vi "Construct Scanner.vi"(11 "Scanner Enum In":T1) -> (0 "error out":errorcluster, 3 "Scanner out":refnum<class "Scanner.lvclass">)   [LabVIEW 2017, in "Scan Driver.lvclass"]
uses:
  Scan Driver.lvclass
  Scanner List.ctl
  Scanners/Scanner/Scanner.lvclass
  Scanners/Dummy Scan/Dummy Scan.lvclass
  C:/LabVIEW-programs/Scanners/Scanner/Scanner.lvclass
  Scanners/Magnetic Field Lakeshore Continuous/Magnetic Field Lakeshore Continuous.lvclass
  Scanners/Magnetic Field Oxford Continuous/Magnetic Field Oxford Continuous.lvclass
  Instruments/Analog Output/Analog Output.lvclass
  Instruments/Function Generator/Function Generator.lvclass
  Instruments/Lakeshore Gaussmeter/Lakeshore Gaussmeter.lvclass
  Instruments/Oxford Magnet/Power Supply/Power Supply.lvclass
  Instruments/Magna-Power Power Supply/Magna Power.lvclass
  Instruments/Microwave/Microwave.lvclass
  Instruments/Pulse Gen/Pulse Generator.lvclass
  Instruments/Translation Stages/Translation Stages.lvclass
  Instruments/Spectrometer/Spectrometer Triax 550.lvclass
  Instruments/Spectrometer ActiveX/Spectrometer ActiveX.lvclass
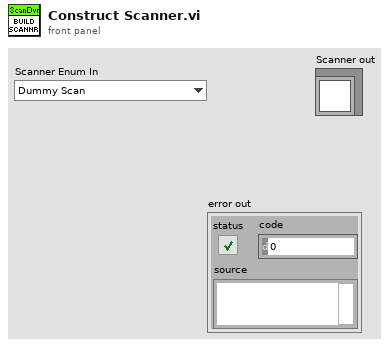
[diagram p1: front panel]
types:
  T1 = typedef "Scan Driver.lvclass/Scanner List.ctl" = enum16{"Dummy Scan", "Analog Output Scan", "Function Gen Scan", "Magnetic Field Lakeshore", "Magnetic Field Lakeshore Continuous", "Magnetic Field Oxford", "Magnetic Field Oxford Continuous", "Magna Current Scan", "Magna Voltage Scan", "Microwave Freq Scan", "Pulse Gen Scan", "Pulse Gen Basic Scan", "Translation Stage Dual", "Translation Stage Coarse", "Translation Stage Fine", "Wavelength", "Wavelength Digikröm", "Wavelength ActiveX", "None"}
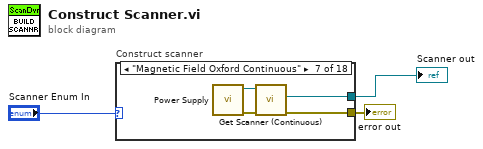
[diagram p0: block diagram]
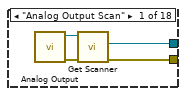
[diagram p2: hidden frame]
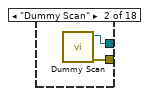
[diagram p3: hidden frame]
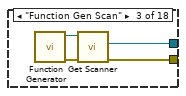
[diagram p4: hidden frame]
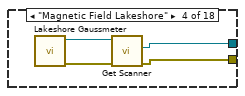
[diagram p5: hidden frame]
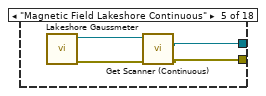
[diagram p6: hidden frame]
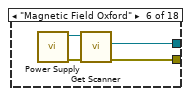
[diagram p7: hidden frame]
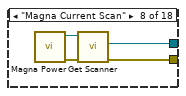
[diagram p8: hidden frame]
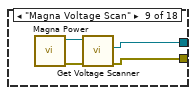
[diagram p9: hidden frame]
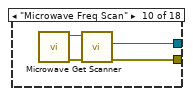
[diagram p10: hidden frame]
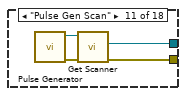
[diagram p11: hidden frame]
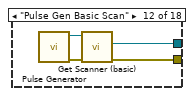
[diagram p12: hidden frame]
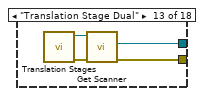
[diagram p13: hidden frame]
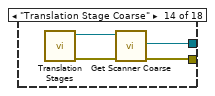
[diagram p14: hidden frame]
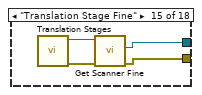
[diagram p15: hidden frame]
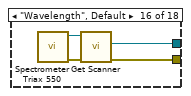
[diagram p16: hidden frame]
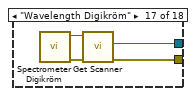
[diagram p17: hidden frame]
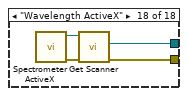
[diagram p18: hidden frame]
diagram:
  n1 = case "Construct scanner" shown="\"Magnetic Field Oxford Continuous\"" "Scanner Enum In" {
    tunnel: [w4 w9 w12 w14 w20 w24 w28 w31 w35 w40 w44 w47 w52 w54 w59 w64 w68 w70] -> w2
    tunnel: [w5 w8 w10 w15 w18 w22 w26 w30 w34 w38 w42 w46 w50 w55 w58 w63 w66 w71] -> w3
    frame "Analog Output Scan" {
      n2 = call "Analog Output.vi"() -> ("error out"=w6:errorcluster, "Analog Output out"=w7:refnum<class "Analog Output.lvclass">)  [unwired: 10 in]
      n3 = call-dynamic "Get Scanner.vi"("error in (no error)"=w6, "Analog Output in"=w7) -> ("error out"=w5:errorcluster, "Default Scanner out"=w4:refnum<class "Scanner.lvclass">)  [unwired: 8 in]
    }
    frame "Dummy Scan" {
      n4 = call "Dummy Scan.vi"() -> ("error out"=w8:errorcluster, "Dummy Scan out"=w9:refnum<class "Dummy Scan.lvclass">)  [unwired: 10 in]
    }
    frame "Function Gen Scan" {
      n5 = call "Function Generator.vi"() -> ("error out"=w11:errorcluster, "Function Generator out"=w13:refnum<class "Function Generator.lvclass">)  [unwired: 1 in, 9 out]
      n6 = call-dynamic "Get Scanner.vi"("error in (no error)"=w11, "Function Generator in"=w13) -> ("error out"=w10:errorcluster, "Default Scanner out"=w12:refnum<class "Scanner.lvclass">)  [unwired: 8 out]
    }
    frame "Magnetic Field Lakeshore" {
      n7 = call "Lakeshore Gaussmeter.vi"() -> ("error out"=w16:errorcluster, "Lakeshore Gaussmeter out"=w17:refnum<class "Lakeshore Gaussmeter.lvclass">)  [unwired: 10 in]
      n8 = call-dynamic "Get Scanner.vi"("error in (no error)"=w16, "Lakeshore Gaussmeter in"=w17) -> ("error out"=w15:errorcluster, "Default Scanner out"=w14:refnum<class "Scanner.lvclass">)  [unwired: 8 in]
    }
    frame "Magnetic Field Lakeshore Continuous" {
      n9 = call "Lakeshore Gaussmeter.vi"() -> ("error out"=w19:errorcluster, "Lakeshore Gaussmeter out"=w21:refnum<class "Lakeshore Gaussmeter.lvclass">)  [unwired: 10 in]
      n10 = call-dynamic "Get Scanner (Continuous).vi"("error in (no error)"=w19, "Lakeshore Gaussmeter in"=w21) -> ("error out"=w18:errorcluster, "Magnetic Field Lakeshore Continuous.lvclass out"=w20:refnum<class "Magnetic Field Lakeshore Continuous.lvclass">)  [unwired: 8 in]
    }
    frame "Magnetic Field Oxford" {
      n11 = call "Power Supply.vi"() -> ("error out"=w23:errorcluster, "Power Supply out"=w25:refnum<class "Power Supply.lvclass">)  [unwired: 10 in]
      n12 = call-dynamic "Get Scanner.vi"("error in (no error)"=w23, "Power Supply in"=w25) -> ("error out"=w22:errorcluster, "Default Scanner out"=w24:refnum<class "Scanner.lvclass">)  [unwired: 8 out]
    }
    frame "Magnetic Field Oxford Continuous" {
      n13 = call "Power Supply.vi"() -> ("error out"=w27:errorcluster, "Power Supply out"=w29:refnum<class "Power Supply.lvclass">)  [unwired: 10 in]
      n14 = call "Get Scanner (Continuous).vi"("error in (no error)"=w27, "Power Supply in"=w29) -> ("error out"=w26:errorcluster, "Continuous Scanner out"=w28:refnum<class "Magnetic Field Oxford Continuous.lvclass">)  [unwired: 8 in]
    }
    frame "Magna Current Scan" {
      n15 = call "Magna Power.vi"() -> ("error out"=w33:errorcluster, "Magna Power out"=w32:refnum<class "Magna Power.lvclass">)  [unwired: 9 in, 1 out]
      n16 = call-dynamic "Get Scanner.vi"("error in (no error)"=w33, "Magna Power in"=w32) -> ("error out"=w30:errorcluster, "Default Scanner out"=w31:refnum<class "Scanner.lvclass">)  [unwired: 8 in]
    }
    frame "Magna Voltage Scan" {
      n17 = call "Magna Power.vi"() -> ("error out"=w37:errorcluster, "Magna Power out"=w36:refnum<class "Magna Power.lvclass">)  [unwired: 9 in, 1 out]
      n18 = call "Get Voltage Scanner.vi"("error in (no error)"=w37, "Magna Power in"=w36) -> ("error out"=w34:errorcluster, "Default Scanner out"=w35:refnum<class "Scanner.lvclass">)  [unwired: 8 in]
    }
    frame "Microwave Freq Scan" {
      n19 = call "Microwave.vi"() -> ("error out"=w39:errorcluster, "Microwave out"=w41:refnum<class "Microwave.lvclass">)  [unwired: 1 in, 9 out]
      n20 = call-dynamic "Get Scanner.vi"("error in (no error)"=w39, "Microwave in"=w41) -> ("error out"=w38:errorcluster, "Default Scanner out"=w40:refnum<class "Scanner.lvclass">)  [unwired: 8 out]
    }
    frame "Pulse Gen Scan" {
      n21 = call "Pulse Generator.vi"() -> ("error out"=w43:errorcluster, "Pulse Generator out"=w45:refnum<class "Pulse Generator.lvclass">)  [unwired: 1 in, 9 out]
      n22 = call-dynamic "Get Scanner.vi"("error in (no error)"=w43, "Pulse Generator in"=w45) -> ("error out"=w42:errorcluster, "Default Scanner out"=w44:refnum<class "Scanner.lvclass">)  [unwired: 8 out]
    }
    frame "Pulse Gen Basic Scan" {
      n23 = call "Pulse Generator.vi"() -> ("error out"=w48:errorcluster, "Pulse Generator out"=w49:refnum<class "Pulse Generator.lvclass">)  [unwired: 1 in, 9 out]
      n24 = call-dynamic "Get Scanner (basic).vi"("error in (no error)"=w48, "Pulse Generator in"=w49) -> ("error out"=w46:errorcluster, "Pulse Gen Basic Scanner out"=w47:refnum<class "Scanner.lvclass">)  [unwired: 8 in]
    }
    frame "Translation Stage Dual" {
      n25 = call "Translation Stages.vi"() -> ("error out"=w51:errorcluster, "Translation Stages out"=w53:refnum<class "Translation Stages.lvclass">)  [unwired: 1 in, 9 out]
      n26 = call-dynamic "Get Scanner.vi"("error in (no error)"=w51, "Translation Stages in"=w53) -> ("error out"=w50:errorcluster, "Default Scanner out"=w52:refnum<class "Scanner.lvclass">)  [unwired: 8 out]
    }
    frame "Translation Stage Coarse" {
      n27 = call "Translation Stages.vi"() -> ("error out"=w56:errorcluster, "Translation Stages out"=w57:refnum<class "Translation Stages.lvclass">)  [unwired: 10 in]
      n28 = call-dynamic "Get Scanner Coarse.vi"("error in (no error)"=w56, "Translation Stages in"=w57) -> ("error out"=w55:errorcluster, "Default Scanner out"=w54:refnum<class "Scanner.lvclass">)  [unwired: 8 in]
    }
    frame "Translation Stage Fine" {
      n29 = call "Translation Stages.vi"() -> ("error out"=w60:errorcluster, "Translation Stages out"=w61:refnum<class "Translation Stages.lvclass">)  [unwired: 10 in]
      n30 = call-dynamic "Get Scanner Fine.vi"("error in (no error)"=w60, "Translation Stages in"=w61) -> ("error out"=w58:errorcluster, "Default Scanner out"=w59:refnum<class "Scanner.lvclass">)  [unwired: 8 in]
    }
    frame "Wavelength", Default {
      n31 = call "Spectrometer Triax 550.vi"() -> ("error out"=w62:errorcluster, "Spectrometer Triax 550 out"=w65:refnum<class "Spectrometer Triax 550.lvclass">)  [unwired: 2 in, 8 out]
      n32 = call-dynamic "Get Scanner.vi"("error in (no error)"=w62, "Spectrometer Triax 550 in"=w65) -> ("error out"=w63:errorcluster, "Default Scanner out"=w64:refnum<class "Scanner.lvclass">)  [unwired: 8 out]
    }
    frame "Wavelength Digikröm" {
      n33 = call "Spectrometer Digikröm.vi"() -> ("error out"=w67:errorcluster, "Spectrometer Digikröm out"=w69:refnum<class "Spectrometer Digikröm.lvclass">)  [unwired: 1 in, 9 out]
      n34 = call-dynamic "Get Scanner.vi"("error in (no error)"=w67, "Spectrometer Digikröm in"=w69) -> ("error out"=w66:errorcluster, "Default Scanner out"=w68:refnum<class "Scanner.lvclass">)  [unwired: 8 out]
    }
    frame "Wavelength ActiveX" {
      n35 = call "Spectrometer ActiveX.vi"() -> ("error out"=w72:errorcluster, "Spectr. iHR320 Out"=w73:refnum<class "Spectrometer ActiveX.lvclass">)  [unwired: 10 in]
      n36 = call-dynamic "Get Scanner.vi"("error in (no error)"=w72, "Spectrometer iHR320 in"=w73) -> ("error out"=w71:errorcluster, "Default Scanner out"=w70:refnum<class "Scanner.lvclass">)  [unwired: 8 in]
    }
  }
  "error out" <- w3
  "Scanner out" <- w2
